vi "To Pretty String (Null).vi"(8 "error in (no error)":errorcluster, 10 "indent":i32) -> (0 "error out":errorcluster, 3 "String":string)   [LabVIEW 2017, in "Advanced Variant Tools.lvlib"]
doc: "Flattens the given JSON data to a string."
uses:
  Advanced Variant Tools.lvlib
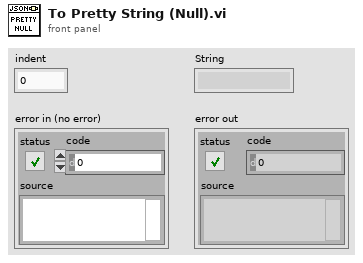
[diagram p1: front panel]
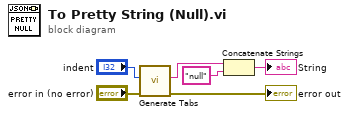
[diagram p0: block diagram]
diagram:
  n1 = call "Generate Tabs.vi"("error in (no error)"="error in (no error)", "indent"="indent") -> ("error out"=→"error out":errorcluster, "Tabs"=w5:string)  [unwired: 8 in]
  n2 = Concatenate Strings(w5, "null" ("String")) -> (→"String":string)
